vi "saturate-detect_fxp16-5.vi"(6 "bound":fxp<+/-,16,5>, 11 "x":fxp<+/-,16,5>) -> (0 "saturated":bool, 2 "sat(x)":fxp<+/-,16,5>)   [LabVIEW 2017]
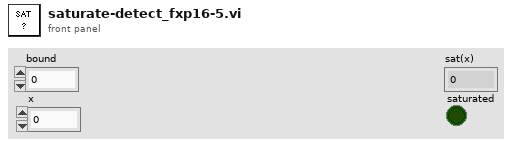
[diagram p1: front panel]
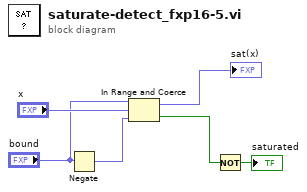
[diagram p0: block diagram]
diagram:
  n1 = Negate(x="bound") -> (-x=w4:fxp<+/-,17,6>)
  n2 = In Range and Coerce(upper limit="bound", x="x", lower limit=w4) -> (coerced(x)=→"sat(x)":fxp<+/-,17,6>, In Range?=w1:bool)
  n3 = Not(x=w1) -> (.not. x?=→"saturated":bool)
